vi "USBL_UA TRACKER for boat_rev2.vi"() -> ()   [LabVIEW 2017]
uses:
  <vilib>/Analysis/2dsp.llb/Decimate (single shot, DBL).vi
  <vilib>/DAQmx/read.llb/DAQmx Read (Analog 1D Wfm NChan NSamp).vi
  <vilib>/Analysis/3filter.llb/FIR Filter (DBL).vi
  <vilib>/DAQmx/create/channels.llb/DAQmx Create Channel (AI-Voltage-Basic).vi
  <vilib>/DAQmx/configure/timing.llb/DAQmx Timing (Sample Clock).vi
  <vilib>/DAQmx/miscellaneous.llb/DAQmx Fill In Error Info.vi
  <vilib>/DAQmx/create/channels.llb/DAQmx Create Channel (CO-Pulse Generation-Frequency).vi
  <vilib>/DAQmx/configure/timing.llb/DAQmx Timing (Implicit).vi
  <vilib>/Analysis/NI_AALBase.lvlib
  <vilib>/Analysis/NI_AALPro.lvlib
  <vilib>/Analysis/NI_AAL_SigProc.lvlib
  <resource>/objmgr/daqmx.rc
panel:
  out "Position 7":dbl[](array[numeric])
  out "Position 6":dbl[](array[numeric])
  out "Position 5":dbl[](array[numeric])
  out "Position 4":dbl[](array[numeric])
  out "Position 3":dbl[](array[numeric])
  out "Position 2":dbl[](array[numeric])
  out "Position 1":dbl[](array[numeric])
  out "Position 0":dbl[](array[numeric])
  out "Deci_Chunk":i32
  out "Target code":dbl[](array[numeric])
  out "ThresholdMargin":dbl=10.0
  out "MovingAvrParm":dbl[](array[numeric])
  out "Coefficient_bit1":dbl[](array[numeric])
  out "Coefficient_bit0":dbl[](array[numeric])
  out "Decimation rate":i32=12
  out "Carrier signal":dbl[](array[numeric])
  out "숫자형 7":dbl=7.0
  out "숫자형 6":dbl=7.0
  out "숫자형 5":dbl=7.0
  in  "Number of pulse":i32=160
  in  "Output terminal":tag="/Dev4/PFI0"
  in  "Frequency(Hz)":dbl=32000.0 format="%.6f"
  in  "Cycle share":dbl=0.5 format="%.6f"
  in  "Counter":tag="Dev4/ctr0"
  out "Detect":bool
  in  "User number":i32=12
  out "숫자형 4":dbl=5.0
  out "숫자형 3":dbl=7.0
  out "숫자형 2":dbl=7.0
  out "숫자형":dbl=7.0
  in  "Start frequency(Hz)":dbl format="%#_6p"
  in  "Stop frequency(Hz)":dbl=4000.0 format="%#_6p"
  in  "Symbol length(sec)":dbl=0.128 format="%#_6p"
  in  "Number of sample":i32=38400
  in  "Sampling freuqncy(Hz)":dbl=192000.0 format="%#_6p"
  in  "Physical channel":tag="Dev4/ai0:7" caption="Physical Channel"
  in  "Device":tag="Dev4"
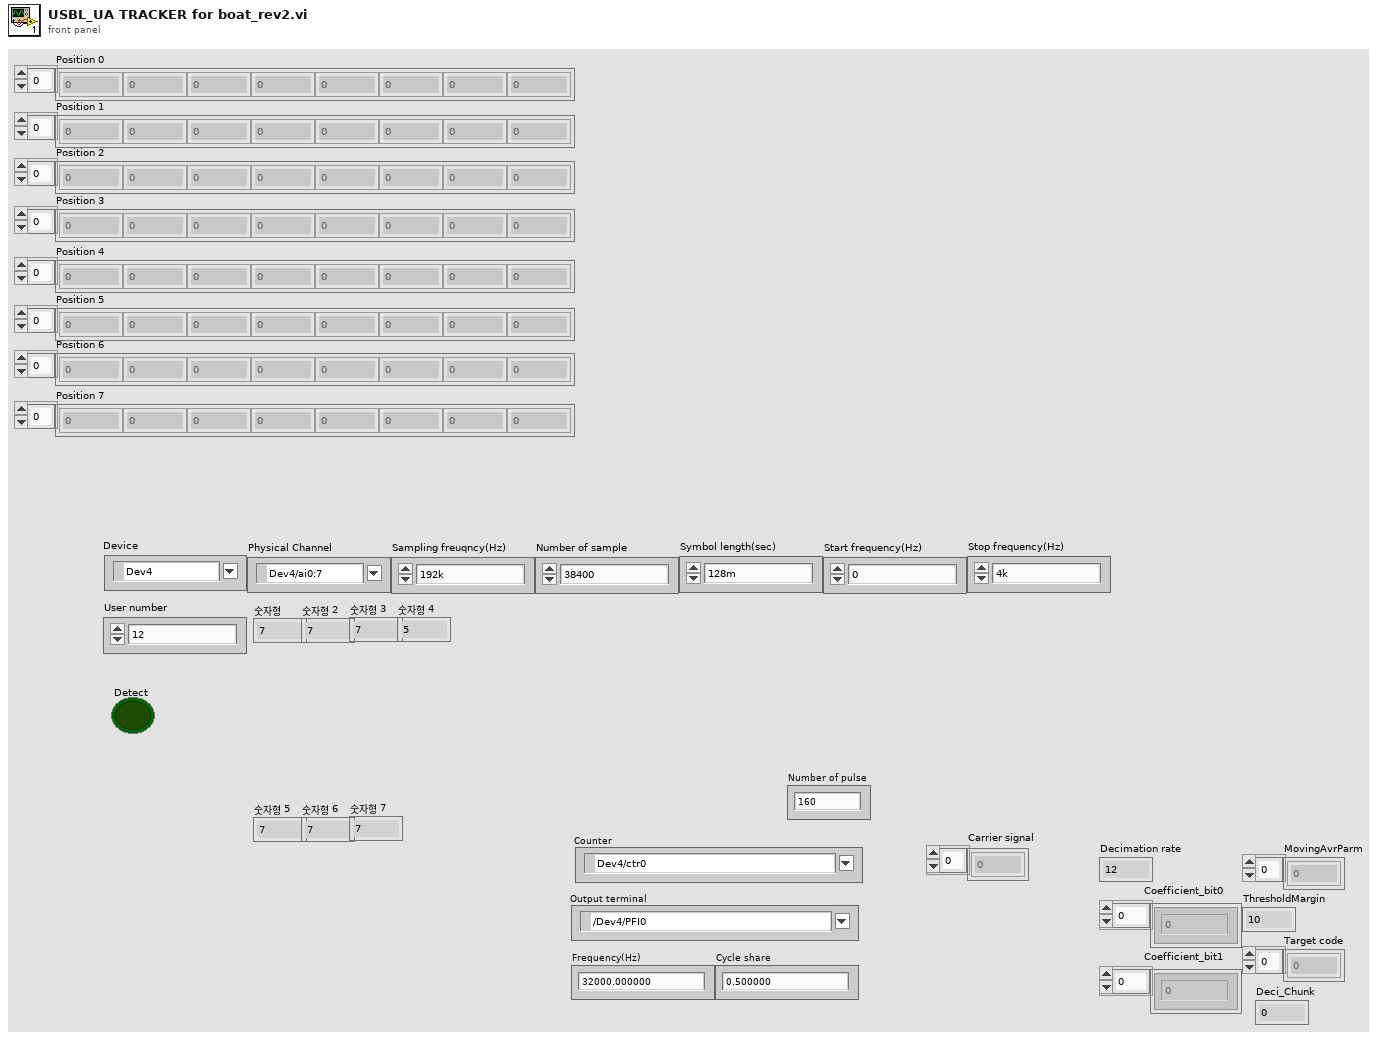
[diagram p1: front panel]
diagram:
  n1 = flat-sequence {
    tunnel: ["Number of sample"] -> w12
    tunnel: [w39] -> w11
    tunnel: ["Sampling freuqncy(Hz)"] -> w10
    tunnel: ["Physical channel"] -> w9
    tunnel: ["Device"] -> w8
    tunnel: [w35] -> w7
    tunnel: [w31] -> w6
    tunnel: [w30] -> w5
    tunnel: [w25] -> w4
    tunnel: [w21] -> w3
    tunnel: [w20] -> w2
    tunnel: [w13] -> w1
    tunnel: w12 -> [w59]
    tunnel: w11 -> [w58]
    tunnel: w10 -> [w57]
    tunnel: w9 -> [w56]
    tunnel: w8 -> [w55]
    tunnel: w7 -> [w54]
    tunnel: w6 -> [w53]
    tunnel: w5 -> [w52]
    tunnel: w4 -> [w49]
    tunnel: w3 -> [w47]
    tunnel: w2 -> [w46]
    tunnel: w1 -> [w43]
    frame #0 {
      w20 = 10.0 ("값")
      w22 = 160 ("차원 크기")
      w35 = 12 ("Divide by")
      w39 = 10123 items=["유한 샘플"=10178, "연속 샘플"=10123, "하드웨어 타이밍에 의한 단일 포인트"=12522] ("sample mode")
      # "Signal gen. (Counter)"
      # "Target code"
      # "EOF"
      # "SOF"
      # "Processing parameter"
      # "Freqeuncy 2"
      # "Freqeuncy 1"
      # "Symbol length"
      # "Moving average window size"
      # "Threshold Margin"
      # "DAQ device setting"
      # "Device"
      # "Physical channel"
      # "Sampling frequency"
      # "Sample mode"
      # "Number of samples per channel"
      n2 = To Double Precision Float(number=w35) -> (double precision float=w41:dbl)
      n3 = To Double Precision Float(number=w22) -> (double precision float=w24:dbl)
      n4 = Divide(x="Sampling freuqncy(Hz)", y=w41) -> (x/y=w29:dbl)
      n5 = Format Into String(format string="%04b" ("포맷 문자열"), "User number") -> (resulting string=w17:string)  [unwired: 2 in, 1 out]
      n6 = Reciprocal(x=w24) -> (1/x=w23:dbl)
      n7 = call "CodeConvert(SubVI).vi"("Code"=w17) -> ("Code_array"=w15:dbl[])
      n8 = Divide(x=30000.0, y="Sampling freuqncy(Hz)") -> (x/y=w33:dbl)
      n9 = Initialize Array(w23, w22) -> (w21:dbl[])
      "MovingAvrParm" <- w21
      n10 = call "ChirpSourceGen(SubVI).vi"("Frequency2(Hz)"="Stop frequency(Hz)", "Frequency1(Hz)"="Start frequency(Hz)", "Pulse length(sec)"="Symbol length(sec)", "Fs(Hz)"=w29) -> ("M.F. Tap(F2-1)"=w25:dbl[], "M.F. Tap(F1-2)"=w31:dbl[])  [unwired: 1 out]
      "Coefficient_bit0" <- w31
      "Coefficient_bit1" <- w25
      n11 = Insert Into Array(array=dbl[] [0.0, 1.0], new element #1=w15, new element #2=dbl[] [1.0, 0.0]) -> (w13:dbl[])  [unwired: 1 in]
      "Target code" <- w13
      n12 = call <vilib>:"Sine Wave.vi"("samples"="Number of sample", "amplitude"=5.0, "frequency"=w33) -> ("sine wave"=w30:dbl[])  [unwired: 2 in, 2 out]
      "Carrier signal" <- w30
      "Decimation rate" <- w35
      "ThresholdMargin" <- w20
    }
    frame #1 {
      n13 = flat-sequence {
        tunnel: w55 -> [w78]
        tunnel: [w79] -> w66
        tunnel: w56 -> [w77]
        tunnel: [w77] -> w65
        tunnel: w57 -> [w75]
        tunnel: [w75] -> w64
        tunnel: w59 -> [w74]
        tunnel: [w74] -> w63
        tunnel: w58 -> [w76]
        tunnel: [w76] -> w62
        tunnel: [w72] -> w61
        tunnel: [w73] -> w60
        tunnel: w54 -> [w73]
        tunnel: w53 -> [w72]
        tunnel: w52 -> [w71]
        tunnel: [w71] -> w51
        tunnel: [w70] -> w50
        tunnel: w49 -> [w70]
        tunnel: [w69] -> w48
        tunnel: w47 -> [w69]
        tunnel: w46 -> [w68]
        tunnel: [w68] -> w45
        tunnel: [w67] -> w44
        tunnel: w43 -> [w67]
        tunnel: w66 -> [w129]
        tunnel: w65 -> [w128]
        tunnel: w64 -> [w127]
        tunnel: w63 -> [w125]
        tunnel: w62 -> [w126]
        tunnel: w61 -> [w114]
        tunnel: w60 -> [w102]
        tunnel: w51 -> [w103]
        tunnel: w50 -> [w87]
        tunnel: w48 -> [w94]
        tunnel: w45 -> [w93]
        tunnel: w44 -> [w88]
        tunnel: [w445] -> w42
        tunnel: w42 -> [w548]
        frame #0 {
          n14 = call <vilib>:"DAQmx Reset Device.vi"("device in"=w78) -> ("error out"=w79:errorcluster)  [unwired: 1 in, 13 out]
        }
        frame #1 {
          w86 = dbl[][] [[-1.0, -1.0, -1.0, -1.0, -1.0, -1.0, -1.0, -1.0], [-1.0, -1.0, -1.0, -1.0, -1.0, -1.0, -1.0, -1.0]]
          w100 = "Proc1" ("이름(이름없음)")
          w101 = "Proc0" ("이름(이름없음)")
          w99 = dbl[][] []
          w115 = "SIG0" ("이름(이름없음)")
          w122 = waveform(dbl) {"t0"=timestamp(0 s since 1904-01-01), "dt"=1.0, "Y"=[]} ("Waveform")
          w105 = "SIG1" ("이름(이름없음)")
          # "Target code"
          # "[Post processing]  1. Queue get : Proc0, Proc1 / 2. Threshold estimation with moving average / 3. Peak and valley detection / 4. Signal detection using time difference of symbol / 5. Demodulation"
          # "[Signal processing]\n1. Queue get : SIG0\n2. Data type converting : Waveform (DBL) --> Array (DBL)\n3. DDC (Digital to Digital Convering)\n  - DSB modulation : Multiply carrier signal (30kHz)\n  - Decimate : 192kHz sample rate --> 16kHz sample rate\n4. Cross-correlation with down-chirp (4k ~ 0Hz)\n5. Envelope detection (Hilbert transform) & square\n6. Queue put : Proc1"
          # "[Signal processing]\n1. Queue get : SIG0\n2. Data type converting : Waveform (DBL) --> Array (DBL)\n3. DDC (Digital to Digital Convering)\n  - DSB modulation : Multiply carrier signal (30kHz)\n  - Decimate : 192kHz sample rate --> 16kHz sample rate\n4. Cross-correlation with up-chirp (0 ~ 4kHz)\n5. Envelope detection (Hilbert transform) & square\n6. Queue put : Proc0"
          # "[Data Acquistion (ADC)]\n1. Device reset\n2. Creat channel\n3, Set sample clock\n  - Sampling frequency : 192kHz\n  - Number of sample (Chunk size) : 38400\n4. Start task\n5. Data read\n6. Queue put : SIG0, SIG1\n  - Queue data type : Waveform (DBL)"
          # "Moving average prameter based on FIR filter calculation"
          # "Coefficient for bit 1 : Down-chirp"
          # "Coefficient for bit 0 : Up-chirp"
          # "Decimation rate"
          # "Carrier signal"
          n15 = call-poly <vilib>:"DAQmx Create Virtual Channel.vi"("physical channels"=w128, "error in"=w129) -> ("task out"=w131:refnum<k21>, "error out"=w130:errorcluster)  [unwired: 7 in, 5 out]
          n16 = call-poly <vilib>:"DAQmx Timing.vi"("task/channels in"=w131, "sample mode"=w126, "samples per channel"=w125, "rate"=w127, "error in"=w130) -> ("task out"=w132:refnum<k21>, "error out"=w133:errorcluster)  [unwired: 2 in, 7 out]
          n17 = call <vilib>:"DAQmx Start Task.vi"("task/channels in"=w132, "error in"=w133) -> ("task out"=w134:refnum<k21>, "error out"=w135:errorcluster)  [unwired: 12 in]
          n18 = Build Array(w122, w122, w122, w122, w122, w122, w122, w122) -> (w104:waveform(dbl)[])
          n19 = Obtain Queue(name (unnamed)=w105, element data type=w104) -> (queue out=w124:refnum<queue>, error out=w123:errorcluster)  [unwired: 3 in, 1 out]
          n20 = Obtain Queue(name (unnamed)=w115, element data type=w104) -> (queue out=w121:refnum<queue>, error out=w120:errorcluster)  [unwired: 3 in, 1 out]
          n21 = while {
            tunnel: w134 -> [w444]
            tunnel: w135 -> [w443]
            tunnel: [w442] -> w138
            tunnel: [w441] -> w139
            tunnel: w125 -> [w440]
            tunnel: w124 -> [w439]
            tunnel: w123 -> [w438]
            tunnel: w121 -> [w437]
            tunnel: w120 -> [w436]
            i -> [w434]
            stop <- w433 stop-if-true
            n22 = call-poly <vilib>:"DAQmx Read.vi"("task/channels in"=w444, "number of samples per channel"=w440, "error in"=w443) -> ("task out"=w442:refnum<k21>, "data"=w435:waveform(dbl)[], "error out"=w441:errorcluster)  [unwired: 10 out]
            n23 = Enqueue Element(queue=w437, element=w435, error in (no error)=w436) -> ()  [unwired: 1 in, 3 out]
            n24 = Enqueue Element(queue=w439, element=w435, error in (no error)=w438) -> ()  [unwired: 1 in, 3 out]
            n25 = local read "Detect"() -> (w433:bool)
            "숫자형" <- w434
          }
          n26 = call <vilib>:"DAQmx Stop Task.vi"("task/channels in"=w138, "error in"=w139) -> ("task out"=w137:refnum<k21>, "error out"=w136:errorcluster)  [unwired: 12 out]
          n27 = call <vilib>:"DAQmx Clear Task.vi"("task in"=w137, "error in"=w136) -> ()  [unwired: 14 out]
          n28 = Obtain Queue(name (unnamed)=w101, element data type=w99) -> (queue out=w119:refnum<queue>, error out=w118:errorcluster)  [unwired: 3 in, 1 out]
          n29 = Obtain Queue(name (unnamed)=w115, element data type=w104) -> (queue out=w117:refnum<queue>, error out=w116:errorcluster)  [unwired: 3 in, 1 out]
          n30 = while {
            tunnel: w117 -> [w432]
            tunnel: w116 -> [w431]
            tunnel: w119 -> [w430]
            tunnel: w118 -> [w429]
            tunnel: [w428] -> w113
            tunnel: [w427] -> w112
            tunnel: w103 -> [w367]
            tunnel: w102 -> [w366]
            tunnel: w114 -> [w365]
            i -> [w363]
            stop <- w362 stop-if-true
            w377 = TRUE ("averaging")
            w426 = TRUE ("init/cont (init:F)")
            n31 = Dequeue Element(queue=w432, error in (no error)=w431) -> (queue out=w428:refnum<queue>, element=w368:waveform(dbl)[], error out=w427:errorcluster)  [unwired: 2 out]
            n32 = Index Array(array=w368) -> (element #1=w425:waveform(dbl), element #2=w424:waveform(dbl), element #3=w423:waveform(dbl), element #4=w422:waveform(dbl), element #5=w421:waveform(dbl), element #6=w420:waveform(dbl), element #7=w419:waveform(dbl), element #8=w418:waveform(dbl))  [unwired: 8 in]
            n33 = Unbundle By Name(w425) -> ("Y"=w417:dbl[])
            n34 = Unbundle By Name(w424) -> ("Y"=w416:dbl[])
            n35 = Unbundle By Name(w423) -> ("Y"=w415:dbl[])
            n36 = Unbundle By Name(w422) -> ("Y"=w414:dbl[])
            n37 = Unbundle By Name(w421) -> ("Y"=w413:dbl[])
            n38 = Unbundle By Name(w420) -> ("Y"=w412:dbl[])
            n39 = Unbundle By Name(w419) -> ("Y"=w411:dbl[])
            n40 = Unbundle By Name(w418) -> ("Y"=w410:dbl[])
            n41 = Multiply(x=w417, y=w367) -> (x*y=w392:dbl[])
            n42 = Multiply(x=w416, y=w367) -> (x*y=w391:dbl[])
            n43 = Multiply(x=w415, y=w367) -> (x*y=w390:dbl[])
            n44 = Multiply(x=w414, y=w367) -> (x*y=w389:dbl[])
            n45 = Multiply(x=w413, y=w367) -> (x*y=w388:dbl[])
            n46 = Multiply(x=w412, y=w367) -> (x*y=w387:dbl[])
            n47 = Multiply(x=w411, y=w367) -> (x*y=w386:dbl[])
            n48 = Multiply(x=w410, y=w367) -> (x*y=w385:dbl[])
            n49 = call-poly <vilib>:"Decimate (single shot).vi"("averaging"=w377, "decimating factor"=w366, "X"=w387) -> ("Decimated Array"=w380:dbl[])  [unwired: 7 in, 1 out]
            n50 = call-poly <vilib>:"Decimate (single shot).vi"("averaging"=w377, "decimating factor"=w366, "X"=w385) -> ("Decimated Array"=w378:dbl[])  [unwired: 7 in, 1 out]
            n51 = call-poly <vilib>:"Decimate (single shot).vi"("averaging"=w377, "decimating factor"=w366, "X"=w391) -> ("Decimated Array"=w384:dbl[])  [unwired: 7 in, 1 out]
            n52 = call-poly <vilib>:"Decimate (single shot).vi"("averaging"=w377, "decimating factor"=w366, "X"=w389) -> ("Decimated Array"=w382:dbl[])  [unwired: 7 in, 1 out]
            n53 = call-poly <vilib>:"Decimate (single shot).vi"("averaging"=w377, "decimating factor"=w366, "X"=w388) -> ("Decimated Array"=w381:dbl[])  [unwired: 7 in, 1 out]
            n54 = call-poly <vilib>:"Decimate (single shot).vi"("averaging"=w377, "decimating factor"=w366, "X"=w386) -> ("Decimated Array"=w379:dbl[])  [unwired: 7 in, 1 out]
            n55 = call-poly <vilib>:"Decimate (single shot).vi"("averaging"=w377, "decimating factor"=w366, "X"=w392) -> ("Decimated Array"=w393:dbl[])  [unwired: 7 in, 1 out]
            n56 = call-poly <vilib>:"Decimate (single shot).vi"("averaging"=w377, "decimating factor"=w366, "X"=w390) -> ("Decimated Array"=w383:dbl[])  [unwired: 7 in, 1 out]
            n57 = call-poly <vilib>:"FIR Filter.vi"("init/cont (init:F)"=w426, "FIR Coefficients"=w365, "X"=w393) -> ("Filtered X"=w409:dbl[])  [unwired: 1 in, 1 out]
            n58 = call-poly <vilib>:"FIR Filter.vi"("init/cont (init:F)"=w426, "FIR Coefficients"=w365, "X"=w384) -> ("Filtered X"=w408:dbl[])  [unwired: 1 in, 1 out]
            n59 = call-poly <vilib>:"FIR Filter.vi"("init/cont (init:F)"=w426, "FIR Coefficients"=w365, "X"=w383) -> ("Filtered X"=w407:dbl[])  [unwired: 1 in, 1 out]
            n60 = call-poly <vilib>:"FIR Filter.vi"("init/cont (init:F)"=w426, "FIR Coefficients"=w365, "X"=w382) -> ("Filtered X"=w406:dbl[])  [unwired: 1 in, 1 out]
            n61 = call-poly <vilib>:"FIR Filter.vi"("init/cont (init:F)"=w426, "FIR Coefficients"=w365, "X"=w381) -> ("Filtered X"=w405:dbl[])  [unwired: 1 in, 1 out]
            n62 = call-poly <vilib>:"FIR Filter.vi"("init/cont (init:F)"=w426, "FIR Coefficients"=w365, "X"=w380) -> ("Filtered X"=w404:dbl[])  [unwired: 1 in, 1 out]
            n63 = call-poly <vilib>:"FIR Filter.vi"("init/cont (init:F)"=w426, "FIR Coefficients"=w365, "X"=w379) -> ("Filtered X"=w403:dbl[])  [unwired: 1 in, 1 out]
            n64 = call-poly <vilib>:"FIR Filter.vi"("init/cont (init:F)"=w426, "FIR Coefficients"=w365, "X"=w378) -> ("Filtered X"=w402:dbl[])  [unwired: 1 in, 1 out]
            n65 = call "Envelope(SubVI).vi"("x"=w409) -> ("Y"=w401:dbl[])
            n66 = call "Envelope(SubVI).vi"("x"=w408) -> ("Y"=w400:dbl[])
            n67 = call "Envelope(SubVI).vi"("x"=w407) -> ("Y"=w399:dbl[])
            n68 = call "Envelope(SubVI).vi"("x"=w406) -> ("Y"=w398:dbl[])
            n69 = call "Envelope(SubVI).vi"("x"=w405) -> ("Y"=w397:dbl[])
            n70 = call "Envelope(SubVI).vi"("x"=w404) -> ("Y"=w396:dbl[])
            n71 = call "Envelope(SubVI).vi"("x"=w403) -> ("Y"=w395:dbl[])
            n72 = call "Envelope(SubVI).vi"("x"=w402) -> ("Y"=w394:dbl[])
            n73 = Square(x=w401) -> (x^2=w376:dbl[])
            n74 = Square(x=w400) -> (x^2=w375:dbl[])
            n75 = Square(x=w399) -> (x^2=w374:dbl[])
            n76 = Square(x=w398) -> (x^2=w373:dbl[])
            n77 = Square(x=w397) -> (x^2=w372:dbl[])
            n78 = Square(x=w396) -> (x^2=w371:dbl[])
            n79 = Square(x=w395) -> (x^2=w370:dbl[])
            n80 = Square(x=w394) -> (x^2=w369:dbl[])
            n81 = local read "Detect"() -> (w362:bool)
            n82 = Build Array(w376, w375, w374, w373, w372, w371, w370, w369) -> (w364:dbl[][])
            n83 = Enqueue Element(queue=w430, element=w364, error in (no error)=w429) -> ()  [unwired: 1 in, 3 out]
            "숫자형 2" <- w363
          }
          n84 = Release Queue(queue=w113, error in (no error)=w112) -> ()  [unwired: 1 in, 3 out]
          n85 = Obtain Queue(name (unnamed)=w100, element data type=w99) -> (queue out=w111:refnum<queue>, error out=w110:errorcluster)  [unwired: 3 in, 1 out]
          n86 = Obtain Queue(name (unnamed)=w105, element data type=w104) -> (queue out=w109:refnum<queue>, error out=w108:errorcluster)  [unwired: 3 in, 1 out]
          n87 = while {
            tunnel: w109 -> [w361]
            tunnel: w108 -> [w360]
            tunnel: w111 -> [w359]
            tunnel: w110 -> [w358]
            tunnel: [w357] -> w107
            tunnel: [w356] -> w106
            tunnel: w103 -> [w296]
            tunnel: w102 -> [w295]
            tunnel: w87 -> [w294]
            i -> [w292]
            stop <- w291 stop-if-true
            w306 = TRUE ("averaging")
            w355 = TRUE ("init/cont (init:F)")
            n88 = Dequeue Element(queue=w361, error in (no error)=w360) -> (queue out=w357:refnum<queue>, element=w297:waveform(dbl)[], error out=w356:errorcluster)  [unwired: 2 out]
            n89 = Index Array(array=w297) -> (element #1=w354:waveform(dbl), element #2=w353:waveform(dbl), element #3=w352:waveform(dbl), element #4=w351:waveform(dbl), element #5=w350:waveform(dbl), element #6=w349:waveform(dbl), element #7=w348:waveform(dbl), element #8=w347:waveform(dbl))  [unwired: 8 in]
            n90 = Unbundle By Name(w354) -> ("Y"=w346:dbl[])
            n91 = Unbundle By Name(w353) -> ("Y"=w345:dbl[])
            n92 = Unbundle By Name(w352) -> ("Y"=w344:dbl[])
            n93 = Unbundle By Name(w351) -> ("Y"=w343:dbl[])
            n94 = Unbundle By Name(w350) -> ("Y"=w342:dbl[])
            n95 = Unbundle By Name(w349) -> ("Y"=w341:dbl[])
            n96 = Unbundle By Name(w348) -> ("Y"=w340:dbl[])
            n97 = Unbundle By Name(w347) -> ("Y"=w339:dbl[])
            n98 = Multiply(x=w346, y=w296) -> (x*y=w321:dbl[])
            n99 = Multiply(x=w345, y=w296) -> (x*y=w320:dbl[])
            n100 = Multiply(x=w344, y=w296) -> (x*y=w319:dbl[])
            n101 = Multiply(x=w343, y=w296) -> (x*y=w318:dbl[])
            n102 = Multiply(x=w342, y=w296) -> (x*y=w317:dbl[])
            n103 = Multiply(x=w341, y=w296) -> (x*y=w316:dbl[])
            n104 = Multiply(x=w340, y=w296) -> (x*y=w315:dbl[])
            n105 = Multiply(x=w339, y=w296) -> (x*y=w314:dbl[])
            n106 = call-poly <vilib>:"Decimate (single shot).vi"("averaging"=w306, "decimating factor"=w295, "X"=w316) -> ("Decimated Array"=w309:dbl[])  [unwired: 7 in, 1 out]
            n107 = call-poly <vilib>:"Decimate (single shot).vi"("averaging"=w306, "decimating factor"=w295, "X"=w314) -> ("Decimated Array"=w307:dbl[])  [unwired: 7 in, 1 out]
            n108 = call-poly <vilib>:"Decimate (single shot).vi"("averaging"=w306, "decimating factor"=w295, "X"=w320) -> ("Decimated Array"=w313:dbl[])  [unwired: 7 in, 1 out]
            n109 = call-poly <vilib>:"Decimate (single shot).vi"("averaging"=w306, "decimating factor"=w295, "X"=w318) -> ("Decimated Array"=w311:dbl[])  [unwired: 7 in, 1 out]
            n110 = call-poly <vilib>:"Decimate (single shot).vi"("averaging"=w306, "decimating factor"=w295, "X"=w317) -> ("Decimated Array"=w310:dbl[])  [unwired: 7 in, 1 out]
            n111 = call-poly <vilib>:"Decimate (single shot).vi"("averaging"=w306, "decimating factor"=w295, "X"=w315) -> ("Decimated Array"=w308:dbl[])  [unwired: 7 in, 1 out]
            n112 = call-poly <vilib>:"Decimate (single shot).vi"("averaging"=w306, "decimating factor"=w295, "X"=w321) -> ("Decimated Array"=w322:dbl[])  [unwired: 7 in, 1 out]
            n113 = call-poly <vilib>:"Decimate (single shot).vi"("averaging"=w306, "decimating factor"=w295, "X"=w319) -> ("Decimated Array"=w312:dbl[])  [unwired: 7 in, 1 out]
            n114 = call-poly <vilib>:"FIR Filter.vi"("init/cont (init:F)"=w355, "FIR Coefficients"=w294, "X"=w322) -> ("Filtered X"=w338:dbl[])  [unwired: 1 in, 1 out]
            n115 = call-poly <vilib>:"FIR Filter.vi"("init/cont (init:F)"=w355, "FIR Coefficients"=w294, "X"=w313) -> ("Filtered X"=w337:dbl[])  [unwired: 1 in, 1 out]
            n116 = call-poly <vilib>:"FIR Filter.vi"("init/cont (init:F)"=w355, "FIR Coefficients"=w294, "X"=w312) -> ("Filtered X"=w336:dbl[])  [unwired: 1 in, 1 out]
            n117 = call-poly <vilib>:"FIR Filter.vi"("init/cont (init:F)"=w355, "FIR Coefficients"=w294, "X"=w311) -> ("Filtered X"=w335:dbl[])  [unwired: 1 in, 1 out]
            n118 = call-poly <vilib>:"FIR Filter.vi"("init/cont (init:F)"=w355, "FIR Coefficients"=w294, "X"=w310) -> ("Filtered X"=w334:dbl[])  [unwired: 1 in, 1 out]
            n119 = call-poly <vilib>:"FIR Filter.vi"("init/cont (init:F)"=w355, "FIR Coefficients"=w294, "X"=w309) -> ("Filtered X"=w333:dbl[])  [unwired: 1 in, 1 out]
            n120 = call-poly <vilib>:"FIR Filter.vi"("init/cont (init:F)"=w355, "FIR Coefficients"=w294, "X"=w308) -> ("Filtered X"=w332:dbl[])  [unwired: 1 in, 1 out]
            n121 = call-poly <vilib>:"FIR Filter.vi"("init/cont (init:F)"=w355, "FIR Coefficients"=w294, "X"=w307) -> ("Filtered X"=w331:dbl[])  [unwired: 1 in, 1 out]
            n122 = call "Envelope(SubVI).vi"("x"=w338) -> ("Y"=w330:dbl[])
            n123 = call "Envelope(SubVI).vi"("x"=w337) -> ("Y"=w329:dbl[])
            n124 = call "Envelope(SubVI).vi"("x"=w336) -> ("Y"=w328:dbl[])
            n125 = call "Envelope(SubVI).vi"("x"=w335) -> ("Y"=w327:dbl[])
            n126 = call "Envelope(SubVI).vi"("x"=w334) -> ("Y"=w326:dbl[])
            n127 = call "Envelope(SubVI).vi"("x"=w333) -> ("Y"=w325:dbl[])
            n128 = call "Envelope(SubVI).vi"("x"=w332) -> ("Y"=w324:dbl[])
            n129 = call "Envelope(SubVI).vi"("x"=w331) -> ("Y"=w323:dbl[])
            n130 = Square(x=w330) -> (x^2=w305:dbl[])
            n131 = Square(x=w329) -> (x^2=w304:dbl[])
            n132 = Square(x=w328) -> (x^2=w303:dbl[])
            n133 = Square(x=w327) -> (x^2=w302:dbl[])
            n134 = Square(x=w326) -> (x^2=w301:dbl[])
            n135 = Square(x=w325) -> (x^2=w300:dbl[])
            n136 = Square(x=w324) -> (x^2=w299:dbl[])
            n137 = Square(x=w323) -> (x^2=w298:dbl[])
            n138 = local read "Detect"() -> (w291:bool)
            n139 = Build Array(w305, w304, w303, w302, w301, w300, w299, w298) -> (w293:dbl[][])
            n140 = Enqueue Element(queue=w359, element=w293, error in (no error)=w358) -> ()  [unwired: 1 in, 3 out]
            "숫자형 3" <- w292
          }
          n141 = local read "Number of sample"() -> (w85:i32)
          n142 = local read "Decimation rate"() -> (w81:i32)
          n143 = To Double Precision Float(number=w81) -> (double precision float=w80:dbl)
          n144 = To Double Precision Float(number=w85) -> (double precision float=w84:dbl)
          n145 = Divide(x=w84, y=w80) -> (x/y=w83:dbl)
          n146 = To Long Integer(number=w83) -> (32bit integer=w82:i32)
          "Deci_Chunk" <- w82
          n147 = Release Queue(queue=w107, error in (no error)=w106) -> ()  [unwired: 1 in, 3 out]
          n148 = Obtain Queue(name (unnamed)=w101, element data type=w99) -> (queue out=w98:refnum<queue>, error out=w97:errorcluster)  [unwired: 3 in, 1 out]
          n149 = Obtain Queue(name (unnamed)=w100, element data type=w99) -> (queue out=w96:refnum<queue>, error out=w95:errorcluster)  [unwired: 3 in, 1 out]
          n150 = while {
            tunnel: w98 -> [w290]
            tunnel: w97 -> [w289]
            tunnel: w96 -> [w288]
            tunnel: w95 -> [w287]
            tunnel: w94 -> [w285]
            tunnel: w93 -> [w249]
            tunnel: [w229] -> w92
            tunnel: [w228] -> w91
            tunnel: [w227] -> w90
            tunnel: [w226] -> w89
            tunnel: w88 -> [w225]
            shift-right: [w140] -> _
            shift-left: w86 -> [w163]
            shift-right: [w141] -> _
            shift-left: w86 -> [w162]
            shift-right: [w142] -> _
            shift-left: w86 -> [w161]
            shift-right: [w143] -> _
            shift-left: w86 -> [w160]
            shift-right: [w144] -> _
            shift-left: w86 -> [w159]
            shift-right: [w145] -> _
            shift-left: w86 -> [w158]
            shift-right: [w146] -> _
            shift-left: w86 -> [w157]
            shift-right: [w147] -> _
            shift-left: w86 -> [w156]
            tunnel: w82 -> [w181]
            i -> [w180]
            stop <- w214 stop-if-true
            w274 = enum32{"Peaks", "Valleys"}."Valleys" ("peaks/valleys")
            w275 = enum32{"Peaks", "Valleys"}."Peaks" ("peaks/valleys")
            w273 = 5 ("width")
            w284 = TRUE ("init/cont (init:F)")
            n151 = Dequeue Element(queue=w290, error in (no error)=w289) -> (queue out=w229:refnum<queue>, element=w231:dbl[][], error out=w228:errorcluster)  [unwired: 2 out]
            n152 = Dequeue Element(queue=w288, error in (no error)=w287) -> (queue out=w227:refnum<queue>, element=w230:dbl[][], error out=w226:errorcluster)  [unwired: 2 out]
            n153 = Subtract(x=w231, y=w230) -> (x-y=w286:dbl[][])
            n154 = Index Array(array=w286) -> (element #1=w272:dbl[], element #2=w271:dbl[], element #3=w270:dbl[], element #4=w269:dbl[], element #5=w268:dbl[], element #6=w267:dbl[], element #7=w266:dbl[], element #8=w234:dbl[])  [unwired: 16 in]
            n155 = call-poly <vilib>:"FIR Filter.vi"("init/cont (init:F)"=w284, "FIR Coefficients"=w285, "X"=w272) -> ("Filtered X"=w283:dbl[])  [unwired: 1 in, 1 out]
            n156 = call-poly <vilib>:"FIR Filter.vi"("init/cont (init:F)"=w284, "FIR Coefficients"=w285, "X"=w271) -> ("Filtered X"=w282:dbl[])  [unwired: 1 in, 1 out]
            n157 = call-poly <vilib>:"FIR Filter.vi"("init/cont (init:F)"=w284, "FIR Coefficients"=w285, "X"=w270) -> ("Filtered X"=w281:dbl[])  [unwired: 1 in, 1 out]
            n158 = call-poly <vilib>:"FIR Filter.vi"("init/cont (init:F)"=w284, "FIR Coefficients"=w285, "X"=w269) -> ("Filtered X"=w280:dbl[])  [unwired: 1 in, 1 out]
            n159 = call-poly <vilib>:"FIR Filter.vi"("init/cont (init:F)"=w284, "FIR Coefficients"=w285, "X"=w268) -> ("Filtered X"=w279:dbl[])  [unwired: 1 in, 1 out]
            n160 = call-poly <vilib>:"FIR Filter.vi"("init/cont (init:F)"=w284, "FIR Coefficients"=w285, "X"=w267) -> ("Filtered X"=w278:dbl[])  [unwired: 1 in, 1 out]
            n161 = call-poly <vilib>:"FIR Filter.vi"("init/cont (init:F)"=w284, "FIR Coefficients"=w285, "X"=w266) -> ("Filtered X"=w277:dbl[])  [unwired: 1 in, 1 out]
            n162 = call-poly <vilib>:"FIR Filter.vi"("init/cont (init:F)"=w284, "FIR Coefficients"=w285, "X"=w234) -> ("Filtered X"=w276:dbl[])  [unwired: 1 in, 1 out]
            n163 = Array Max & Min(array=w283) -> (max value=w265:dbl, min value=w264:dbl)  [unwired: 2 out]
            n164 = Array Max & Min(array=w282) -> (max value=w263:dbl, min value=w262:dbl)  [unwired: 2 out]
            n165 = Array Max & Min(array=w281) -> (max value=w261:dbl, min value=w260:dbl)  [unwired: 2 out]
            n166 = Array Max & Min(array=w280) -> (max value=w259:dbl, min value=w258:dbl)  [unwired: 2 out]
            n167 = Array Max & Min(array=w279) -> (max value=w257:dbl, min value=w256:dbl)  [unwired: 2 out]
            n168 = Array Max & Min(array=w278) -> (max value=w255:dbl, min value=w254:dbl)  [unwired: 2 out]
            n169 = Array Max & Min(array=w277) -> (max value=w253:dbl, min value=w252:dbl)  [unwired: 2 out]
            n170 = Array Max & Min(array=w276) -> (max value=w251:dbl, min value=w250:dbl)  [unwired: 2 out]
            n171 = call "ThresholdEstimation(SubVI).vi"("Margin"=w249, "최소값"=w262, "최대값"=w263) -> ("N.Th"=w236:dbl, "P.Th"=w247:dbl)
            n172 = call "ThresholdEstimation(SubVI).vi"("Margin"=w249, "최소값"=w260, "최대값"=w261) -> ("N.Th"=w237:dbl, "P.Th"=w246:dbl)
            n173 = call "ThresholdEstimation(SubVI).vi"("Margin"=w249, "최소값"=w258, "최대값"=w259) -> ("N.Th"=w238:dbl, "P.Th"=w245:dbl)
            n174 = call "ThresholdEstimation(SubVI).vi"("Margin"=w249, "최소값"=w256, "최대값"=w257) -> ("N.Th"=w239:dbl, "P.Th"=w244:dbl)
            n175 = call "ThresholdEstimation(SubVI).vi"("Margin"=w249, "최소값"=w264, "최대값"=w265) -> ("N.Th"=w235:dbl, "P.Th"=w248:dbl)
            n176 = call "ThresholdEstimation(SubVI).vi"("Margin"=w249, "최소값"=w254, "최대값"=w255) -> ("N.Th"=w240:dbl, "P.Th"=w243:dbl)
            n177 = call "ThresholdEstimation(SubVI).vi"("Margin"=w249, "최소값"=w252, "최대값"=w253) -> ("N.Th"=w241:dbl, "P.Th"=w242:dbl)
            n178 = call "ThresholdEstimation(SubVI).vi"("Margin"=w249, "최소값"=w250, "최대값"=w251) -> ("N.Th"=w233:dbl, "P.Th"=w232:dbl)
            n179 = call <vilib>:"Peak Detector.vi"("peaks/valleys"=w275, "width"=w273, "threshold"=w248, "X"=w272) -> ("Locations"=w211:dbl[], "# found"=w213:i32)  [unwired: 3 in, 3 out]
            n180 = call <vilib>:"Peak Detector.vi"("peaks/valleys"=w275, "width"=w273, "threshold"=w247, "X"=w271) -> ("Locations"=w207:dbl[], "# found"=w209:i32)  [unwired: 3 in, 3 out]
            n181 = call <vilib>:"Peak Detector.vi"("peaks/valleys"=w275, "width"=w273, "threshold"=w246, "X"=w270) -> ("Locations"=w203:dbl[], "# found"=w205:i32)  [unwired: 3 in, 3 out]
            n182 = call <vilib>:"Peak Detector.vi"("peaks/valleys"=w275, "width"=w273, "threshold"=w245, "X"=w269) -> ("Locations"=w199:dbl[], "# found"=w201:i32)  [unwired: 3 in, 3 out]
            n183 = call <vilib>:"Peak Detector.vi"("peaks/valleys"=w275, "width"=w273, "threshold"=w244, "X"=w268) -> ("Locations"=w195:dbl[], "# found"=w197:i32)  [unwired: 3 in, 3 out]
            n184 = call <vilib>:"Peak Detector.vi"("peaks/valleys"=w275, "width"=w273, "threshold"=w243, "X"=w267) -> ("Locations"=w191:dbl[], "# found"=w193:i32)  [unwired: 3 in, 3 out]
            n185 = call <vilib>:"Peak Detector.vi"("peaks/valleys"=w275, "width"=w273, "threshold"=w242, "X"=w266) -> ("Locations"=w187:dbl[], "# found"=w189:i32)  [unwired: 3 in, 3 out]
            n186 = call <vilib>:"Peak Detector.vi"("peaks/valleys"=w275, "width"=w273, "threshold"=w232, "X"=w234) -> ("Locations"=w183:dbl[], "# found"=w185:i32)  [unwired: 3 in, 3 out]
            n187 = call <vilib>:"Peak Detector.vi"("peaks/valleys"=w274, "width"=w273, "threshold"=w235, "X"=w272) -> ("Locations"=w210:dbl[], "# found"=w212:i32)  [unwired: 3 in, 3 out]
            n188 = call <vilib>:"Peak Detector.vi"("peaks/valleys"=w274, "width"=w273, "threshold"=w236, "X"=w271) -> ("Locations"=w206:dbl[], "# found"=w208:i32)  [unwired: 3 in, 3 out]
            n189 = call <vilib>:"Peak Detector.vi"("peaks/valleys"=w274, "width"=w273, "threshold"=w237, "X"=w270) -> ("Locations"=w202:dbl[], "# found"=w204:i32)  [unwired: 3 in, 3 out]
            n190 = call <vilib>:"Peak Detector.vi"("peaks/valleys"=w274, "width"=w273, "threshold"=w238, "X"=w269) -> ("Locations"=w198:dbl[], "# found"=w200:i32)  [unwired: 3 in, 3 out]
            n191 = call <vilib>:"Peak Detector.vi"("peaks/valleys"=w274, "width"=w273, "threshold"=w239, "X"=w268) -> ("Locations"=w194:dbl[], "# found"=w196:i32)  [unwired: 3 in, 3 out]
            n192 = call <vilib>:"Peak Detector.vi"("peaks/valleys"=w274, "width"=w273, "threshold"=w240, "X"=w267) -> ("Locations"=w190:dbl[], "# found"=w192:i32)  [unwired: 3 in, 3 out]
            n193 = call <vilib>:"Peak Detector.vi"("peaks/valleys"=w274, "width"=w273, "threshold"=w241, "X"=w266) -> ("Locations"=w186:dbl[], "# found"=w188:i32)  [unwired: 3 in, 3 out]
            n194 = call <vilib>:"Peak Detector.vi"("peaks/valleys"=w274, "width"=w273, "threshold"=w233, "X"=w234) -> ("Locations"=w182:dbl[], "# found"=w184:i32)  [unwired: 3 in, 3 out]
            n195 = call "Decision2(SubVI).vi"("L_ind0"=w213, "number of sample"=w181, "L_ind1"=w212, "Peak_ind0"=w211, "index"=w180, "Peak_ind1"=w210) -> ("L_sum"=w148:i32, "Bits"=w179:dbl[], "Position"=w178:dbl[])
            n196 = call "Decision2(SubVI).vi"("L_ind0"=w209, "number of sample"=w181, "L_ind1"=w208, "Peak_ind0"=w207, "index"=w180, "Peak_ind1"=w206) -> ("L_sum"=w149:i32, "Bits"=w177:dbl[], "Position"=w176:dbl[])
            n197 = call "Decision2(SubVI).vi"("L_ind0"=w205, "number of sample"=w181, "L_ind1"=w204, "Peak_ind0"=w203, "index"=w180, "Peak_ind1"=w202) -> ("L_sum"=w150:i32, "Bits"=w175:dbl[], "Position"=w174:dbl[])
            n198 = call "Decision2(SubVI).vi"("L_ind0"=w201, "number of sample"=w181, "L_ind1"=w200, "Peak_ind0"=w199, "index"=w180, "Peak_ind1"=w198) -> ("L_sum"=w151:i32, "Bits"=w173:dbl[], "Position"=w172:dbl[])
            n199 = call "Decision2(SubVI).vi"("L_ind0"=w197, "number of sample"=w181, "L_ind1"=w196, "Peak_ind0"=w195, "index"=w180, "Peak_ind1"=w194) -> ("L_sum"=w152:i32, "Bits"=w171:dbl[], "Position"=w170:dbl[])
            n200 = call "Decision2(SubVI).vi"("L_ind0"=w193, "number of sample"=w181, "L_ind1"=w192, "Peak_ind0"=w191, "index"=w180, "Peak_ind1"=w190) -> ("L_sum"=w153:i32, "Bits"=w169:dbl[], "Position"=w168:dbl[])
            n201 = call "Decision2(SubVI).vi"("L_ind0"=w189, "number of sample"=w181, "L_ind1"=w188, "Peak_ind0"=w187, "index"=w180, "Peak_ind1"=w186) -> ("L_sum"=w154:i32, "Bits"=w167:dbl[], "Position"=w166:dbl[])
            n202 = call "Decision2(SubVI).vi"("L_ind0"=w185, "number of sample"=w181, "L_ind1"=w184, "Peak_ind0"=w183, "index"=w180, "Peak_ind1"=w182) -> ("L_sum"=w155:i32, "Bits"=w165:dbl[], "Position"=w164:dbl[])
            n203 = call "TImeThresholdLogic(SubVI).vi"("Position"=w178, "Bits"=w179, "Buffer"=w163) -> ("Data"=w140:dbl[][])  [unwired: 1 in]
            n204 = call "TImeThresholdLogic(SubVI).vi"("Position"=w176, "Bits"=w177, "Buffer"=w162) -> ("Data"=w141:dbl[][])  [unwired: 1 in]
            n205 = call "TImeThresholdLogic(SubVI).vi"("Position"=w174, "Bits"=w175, "Buffer"=w161) -> ("Data"=w142:dbl[][])  [unwired: 1 in]
            n206 = call "TImeThresholdLogic(SubVI).vi"("Position"=w172, "Bits"=w173, "Buffer"=w160) -> ("Data"=w143:dbl[][])  [unwired: 1 in]
            n207 = call "TImeThresholdLogic(SubVI).vi"("Position"=w170, "Bits"=w171, "Buffer"=w159) -> ("Data"=w144:dbl[][])  [unwired: 1 in]
            n208 = call "TImeThresholdLogic(SubVI).vi"("Position"=w168, "Bits"=w169, "Buffer"=w158) -> ("Data"=w145:dbl[][])  [unwired: 1 in]
            n209 = call "TImeThresholdLogic(SubVI).vi"("Position"=w166, "Bits"=w167, "Buffer"=w157) -> ("Data"=w146:dbl[][])  [unwired: 1 in]
            n210 = call "TImeThresholdLogic(SubVI).vi"("Position"=w164, "Bits"=w165, "Buffer"=w156) -> ("Data"=w147:dbl[][])  [unwired: 1 in]
            n211 = call "CodeDetection(SubVI).vi"("Code"=w225, "Buff"=w140, "L_sum"=w148) -> ("detect"=w224:bool)  [unwired: 1 out]
            n212 = call "CodeDetection(SubVI).vi"("Code"=w225, "Buff"=w141, "L_sum"=w149) -> ("detect"=w223:bool)  [unwired: 1 out]
            n213 = call "CodeDetection(SubVI).vi"("Code"=w225, "Buff"=w142, "L_sum"=w150) -> ("detect"=w222:bool)  [unwired: 1 out]
            n214 = call "CodeDetection(SubVI).vi"("Code"=w225, "Buff"=w143, "L_sum"=w151) -> ("detect"=w221:bool)  [unwired: 1 out]
            n215 = call "CodeDetection(SubVI).vi"("Code"=w225, "Buff"=w144, "L_sum"=w152) -> ("detect"=w220:bool)  [unwired: 1 out]
            n216 = call "CodeDetection(SubVI).vi"("Code"=w225, "Buff"=w145, "L_sum"=w153) -> ("detect"=w219:bool)  [unwired: 1 out]
            n217 = call "CodeDetection(SubVI).vi"("Code"=w225, "Buff"=w146, "L_sum"=w154) -> ("detect"=w218:bool)  [unwired: 1 out]
            n218 = call "CodeDetection(SubVI).vi"("Code"=w225, "Buff"=w147, "L_sum"=w155) -> ("detect"=w217:bool)  [unwired: 1 out]
            n219 = Build Array(w224, w223, w222, w221, w220, w219, w218, w217) -> (w216:bool[])
            n220 = Boolean Array To Number(Boolean array=w216) -> (number=w215:u32)
            n221 = Greater Than 0?(x=w215) -> (x > 0?=w214:bool)
            "Detect" <- w214
            "숫자형 4" <- w180
          }
          n222 = Release Queue(queue=w92, error in (no error)=w91) -> ()  [unwired: 1 in, 3 out]
          n223 = Release Queue(queue=w90, error in (no error)=w89) -> ()  [unwired: 1 in, 3 out]
        }
        frame #2 {
          n224 = local read "Device"() -> (w446:tag)
          n225 = call <vilib>:"DAQmx Reset Device.vi"("device in"=w446) -> ("error out"=w445:errorcluster)  [unwired: 1 in, 13 out]
        }
        frame #3 {
          w447 = dbl[] []
          w456 = dbl[][] [[-1.0, -1.0, -1.0, -1.0, -1.0, -1.0, -1.0, -1.0], [-1.0, -1.0, -1.0, -1.0, -1.0, -1.0, -1.0, -1.0]]
          w475 = dbl[][] []
          w491 = waveform(dbl) {"t0"=timestamp(0 s since 1904-01-01), "dt"=1.0, "Y"=[]} ("Waveform")
          w468 = "Proc1" ("이름(이름없음)")
          w467 = "Proc0" ("이름(이름없음)")
          w466 = dbl[][] []
          w514 = "SIG0" ("이름(이름없음)")
          w521 = waveform(dbl) {"t0"=timestamp(0 s since 1904-01-01), "dt"=1.0, "Y"=[]} ("Waveform")
          w505 = "SIG1" ("이름(이름없음)")
          w537 = 10123 items=["유한 샘플"=10178, "연속 샘플"=10123, "하드웨어 타이밍에 의한 단일 포인트"=12522] ("sample mode")
          w541 = 10178 items=["유한 샘플"=10178, "연속 샘플"=10123, "하드웨어 타이밍에 의한 단일 포인트"=12522] ("sample mode")
          # "[Post processing]  1. Queue get : Proc0, Proc1 / 2. Threshold estimation with moving average / 3. Peak and valley detection / 4. Demodulation"
          # "[Rx.time]\nTravel time (1km) : 670ms * 2\nDown-link : 210ms\nUp-link : 1024ms\nTotal : Rx.time > 2574ms"
          # "Local variable"
          # "Queue clear"
          # "[Data Acquistion (ADC)]"
          # "Signal generation (Counter) / delaty time : 200ms"
          # "[Signal processing]\n1. Queue get : SIG0\n2. Data type converting : Waveform (DBL) --> Array (DBL)\n3. DDC (Digital to Digital Convering)\n  - DSB modulation : Multiply carrier signal (30kHz)\n  - Decimate : 192kHz sample rate --> 16kHz sample rate\n4. Cross-correlation with down-chirp (4k ~ 0Hz)\n5. Envelope detection (Hilbert transform) & square\n6. Queue put : Proc1"
          # "[Signal processing]\n1. Queue get : SIG0\n2. Data type converting : Waveform (DBL) --> Array (DBL)\n3. DDC (Digital to Digital Convering)\n  - DSB modulation : Multiply carrier signal (30kHz)\n  - Decimate : 192kHz sample rate --> 16kHz sample rate\n4. Cross-correlation with up-chirp (0 ~ 4kHz)\n5. Envelope detection (Hilbert transform) & square\n6. Queue put : Proc0"
          # "[Data Acquistion (ADC)]\n1. Device reset\n2. Creat channel\n3, Set sample clock\n  - Sampling frequency : 192kHz\n  - Number of sample (Chunk size) : 38400\n4. Start task\n5. Data read\n6. Queue put : SIG0, SIG1\n  - Queue data type : Waveform (DBL)"
          n226 = local read "Number of pulse"() -> (w542:i32)
          n227 = local read "Output terminal"() -> (w545:tag)
          n228 = local read "Sampling freuqncy(Hz)"() -> (w473:dbl)
          n229 = local read "Physical channel"() -> (w539:tag)
          n230 = local read "Frequency(Hz)"() -> (w550:dbl)
          n231 = Build Array(w491, w491, w491, w491, w491, w491, w491, w491) -> (w490:waveform(dbl)[])
          n232 = local read "Cycle share"() -> (w549:dbl)
          n233 = local read "Number of sample"() -> (w472:i32)
          n234 = local read "Counter"() -> (w551:tag)
          n235 = Obtain Queue(name (unnamed)="SIG1" ("이름(이름없음)"), element data type=w490) -> (queue out=w487:refnum<queue>, error out=w486:errorcluster)  [unwired: 3 in, 1 out]
          n236 = Obtain Queue(name (unnamed)="Proc1" ("이름(이름없음)"), element data type=w475) -> (queue out=w479:refnum<queue>, error out=w478:errorcluster)  [unwired: 3 in, 1 out]
          n237 = Obtain Queue(name (unnamed)="SIG0" ("이름(이름없음)"), element data type=w490) -> (queue out=w497:refnum<queue>, error out=w496:errorcluster)  [unwired: 3 in, 1 out]
          n238 = Obtain Queue(name (unnamed)="Proc0" ("이름(이름없음)"), element data type=w475) -> (queue out=w485:refnum<queue>, error out=w484:errorcluster)  [unwired: 3 in, 1 out]
          n239 = call-poly <vilib>:"DAQmx Create Virtual Channel.vi"("frequency"=w550, "duty cycle"=w549, "counter"=w551, "error in"=w548) -> ("task out"=w547:refnum<k21>, "error out"=w546:errorcluster)  [unwired: 10 in]
          n240 = call-poly <vilib>:"DAQmx Create Virtual Channel.vi"("physical channels"=w539) -> ("task out"=w538:refnum<k21>, "error out"=w540:errorcluster)  [unwired: 8 in, 5 out]
          n241 = Flush Queue(queue=w497, error in (no error)=w496) -> (queue out=w495:refnum<queue>, error out=w494:errorcluster)  [unwired: 1 out]
          n242 = Flush Queue(queue=w487, error in (no error)=w486) -> (queue out=w489:refnum<queue>, error out=w488:errorcluster)  [unwired: 1 out]
          n243 = Flush Queue(queue=w485, error in (no error)=w484) -> (queue out=w483:refnum<queue>, error out=w482:errorcluster)  [unwired: 1 out]
          n244 = Flush Queue(queue=w479, error in (no error)=w478) -> (queue out=w481:refnum<queue>, error out=w480:errorcluster)  [unwired: 1 out]
          n245 = property class="DAQmx 채널"(reference=w547, error in=w546, "CO.Pulse.Term"=w545) -> (reference out=w544:refnum<k21>, error out=w543:errorcluster)
          n246 = Release Queue(queue=w495, error in (no error)=w494) -> ()  [unwired: 1 in, 3 out]
          n247 = Release Queue(queue=w489, error in (no error)=w488) -> ()  [unwired: 1 in, 3 out]
          n248 = Release Queue(queue=w483, error in (no error)=w482) -> ()  [unwired: 1 in, 3 out]
          n249 = Release Queue(queue=w481, error in (no error)=w480) -> ()  [unwired: 1 in, 3 out]
          n250 = call-poly <vilib>:"DAQmx Timing.vi"("task/channels in"=w538, "sample mode"=w537, "samples per channel"=w472, "rate"=w473, "error in"=w540) -> ("task out"=w536:refnum<k21>, "error out"=w535:errorcluster)  [unwired: 2 in, 7 out]
          n251 = call-poly <vilib>:"DAQmx Timing.vi"("task/channels in"=w544, "sample mode"=w541, "samples per channel"=w542, "error in"=w543) -> ("task out"=w534:refnum<k21>, "error out"=w533:errorcluster)  [unwired: 10 in]
          n252 = flat-sequence {
            tunnel: w536 -> [w889]
            tunnel: w535 -> [w888]
            tunnel: w534 -> [w887]
            tunnel: w533 -> [w886]
            tunnel: [w887] -> w532
            tunnel: [w886] -> w531
            tunnel: [w885] -> w503
            tunnel: [w884] -> w502
            frame #0 {
              n253 = call <vilib>:"DAQmx Start Task.vi"("task/channels in"=w889, "error in"=w888) -> ("task out"=w885:refnum<k21>, "error out"=w884:errorcluster)  [unwired: 12 in]
            }
          }
          n254 = for {
            N: 2 -> [_]
            tunnel: w532 -> [w882]
            tunnel: [w877] -> w529
            tunnel: w531 -> [w883]
            tunnel: [w876] -> w528
            n255 = call <vilib>:"DAQmx Start Task.vi"("task/channels in"=w882, "error in"=w883) -> ("task out"=w881:refnum<k21>, "error out"=w880:errorcluster)  [unwired: 12 in]
            n256 = call <vilib>:"DAQmx Is Task Done.vi"("task/channels in"=w881, "error in"=w880) -> ("task out"=w879:refnum<k21>, "error out"=w878:errorcluster)  [unwired: 11 in, 1 out]
            n257 = Wait (ms)(milliseconds to wait=u32 200 ("대기 시간 (ms)")) -> ()  [unwired: 1 out]
            n258 = call <vilib>:"DAQmx Stop Task.vi"("task/channels in"=w879, "error in"=w878) -> ("task out"=w877:refnum<k21>, "error out"=w876:errorcluster)  [unwired: 12 in]
          }
          n259 = Multiply(x=3.0, y=w473) -> (x*y=w471:dbl)
          n260 = To Double Precision Float(number=w472) -> (double precision float=w470:dbl)
          n261 = Divide(x=w471, y=w470) -> (x/y=w469:dbl)
          n262 = To Long Integer(number=w469) -> (32bit integer=w457:i32)
          n263 = call <vilib>:"DAQmx Clear Task.vi"("task in"=w529, "error in"=w528) -> ()  [unwired: 13 in, 1 out]
          n264 = Build Array(w521, w521, w521, w521, w521, w521, w521, w521) -> (w504:waveform(dbl)[])
          n265 = Obtain Queue(name (unnamed)=w505, element data type=w504) -> (queue out=w523:refnum<queue>, error out=w522:errorcluster)  [unwired: 3 in, 1 out]
          n266 = Obtain Queue(name (unnamed)=w514, element data type=w504) -> (queue out=w520:refnum<queue>, error out=w519:errorcluster)  [unwired: 3 in, 1 out]
          n267 = for {
            N: w457 -> [_]
            tunnel: w503 -> [w874]
            tunnel: w502 -> [w873]
            tunnel: [w872] -> w526
            tunnel: [w871] -> w527
            tunnel: w472 -> [w870]
            tunnel: w523 -> [w869]
            tunnel: w522 -> [w868]
            tunnel: w520 -> [w867]
            tunnel: w519 -> [w866]
            i -> [w864]
            n268 = call-poly <vilib>:"DAQmx Read.vi"("task/channels in"=w874, "number of samples per channel"=w870, "error in"=w873) -> ("task out"=w872:refnum<k21>, "data"=w865:waveform(dbl)[], "error out"=w871:errorcluster)  [unwired: 10 out]
            n269 = Enqueue Element(queue=w867, element=w865, error in (no error)=w866) -> ()  [unwired: 1 in, 3 out]
            n270 = Enqueue Element(queue=w869, element=w865, error in (no error)=w868) -> ()  [unwired: 1 in, 3 out]
            "숫자형 5" <- w864
          }
          n271 = local read "Decimation rate"() -> (w500:i32)
          n272 = local read "Coefficient_bit0"() -> (w499:dbl[])
          n273 = local read "Coefficient_bit1"() -> (w498:dbl[])
          n274 = local read "MovingAvrParm"() -> (w461:dbl[])
          n275 = local read "ThresholdMargin"() -> (w460:dbl)
          n276 = local read "Deci_Chunk"() -> (w459:i32)
          n277 = local read "Target code"() -> (w458:dbl[])
          n278 = local read "Carrier signal"() -> (w501:dbl[])
          n279 = call <vilib>:"DAQmx Stop Task.vi"("task/channels in"=w526, "error in"=w527) -> ("task out"=w525:refnum<k21>, "error out"=w524:errorcluster)  [unwired: 12 out]
          n280 = call <vilib>:"DAQmx Clear Task.vi"("task in"=w525, "error in"=w524) -> ()  [unwired: 14 out]
          n281 = Obtain Queue(name (unnamed)=w467, element data type=w466) -> (queue out=w518:refnum<queue>, error out=w517:errorcluster)  [unwired: 3 in, 1 out]
          n282 = Obtain Queue(name (unnamed)=w514, element data type=w504) -> (queue out=w516:refnum<queue>, error out=w515:errorcluster)  [unwired: 3 in, 1 out]
          n283 = for {
            N: w457 -> [_]
            tunnel: w516 -> [w863]
            tunnel: w515 -> [w862]
            tunnel: w518 -> [w861]
            tunnel: w517 -> [w860]
            tunnel: [w859] -> w513
            tunnel: [w858] -> w512
            tunnel: w501 -> [w798]
            tunnel: w500 -> [w797]
            tunnel: w499 -> [w796]
            i -> [w794]
            w808 = TRUE ("averaging")
            w857 = TRUE ("init/cont (init:F)")
            n284 = Dequeue Element(queue=w863, error in (no error)=w862) -> (queue out=w859:refnum<queue>, element=w799:waveform(dbl)[], error out=w858:errorcluster)  [unwired: 2 out]
            n285 = Index Array(array=w799) -> (element #1=w856:waveform(dbl), element #2=w855:waveform(dbl), element #3=w854:waveform(dbl), element #4=w853:waveform(dbl), element #5=w852:waveform(dbl), element #6=w851:waveform(dbl), element #7=w850:waveform(dbl), element #8=w849:waveform(dbl))  [unwired: 8 in]
            n286 = Unbundle By Name(w856) -> ("Y"=w848:dbl[])
            n287 = Unbundle By Name(w855) -> ("Y"=w847:dbl[])
            n288 = Unbundle By Name(w854) -> ("Y"=w846:dbl[])
            n289 = Unbundle By Name(w853) -> ("Y"=w845:dbl[])
            n290 = Unbundle By Name(w852) -> ("Y"=w844:dbl[])
            n291 = Unbundle By Name(w851) -> ("Y"=w843:dbl[])
            n292 = Unbundle By Name(w850) -> ("Y"=w842:dbl[])
            n293 = Unbundle By Name(w849) -> ("Y"=w841:dbl[])
            n294 = Multiply(x=w848, y=w798) -> (x*y=w823:dbl[])
            n295 = Multiply(x=w847, y=w798) -> (x*y=w822:dbl[])
            n296 = Multiply(x=w846, y=w798) -> (x*y=w821:dbl[])
            n297 = Multiply(x=w845, y=w798) -> (x*y=w820:dbl[])
            n298 = Multiply(x=w844, y=w798) -> (x*y=w819:dbl[])
            n299 = Multiply(x=w843, y=w798) -> (x*y=w818:dbl[])
            n300 = Multiply(x=w842, y=w798) -> (x*y=w817:dbl[])
            n301 = Multiply(x=w841, y=w798) -> (x*y=w816:dbl[])
            n302 = call-poly <vilib>:"Decimate (single shot).vi"("averaging"=w808, "decimating factor"=w797, "X"=w818) -> ("Decimated Array"=w811:dbl[])  [unwired: 7 in, 1 out]
            n303 = call-poly <vilib>:"Decimate (single shot).vi"("averaging"=w808, "decimating factor"=w797, "X"=w816) -> ("Decimated Array"=w809:dbl[])  [unwired: 7 in, 1 out]
            n304 = call-poly <vilib>:"Decimate (single shot).vi"("averaging"=w808, "decimating factor"=w797, "X"=w822) -> ("Decimated Array"=w815:dbl[])  [unwired: 7 in, 1 out]
            n305 = call-poly <vilib>:"Decimate (single shot).vi"("averaging"=w808, "decimating factor"=w797, "X"=w820) -> ("Decimated Array"=w813:dbl[])  [unwired: 7 in, 1 out]
            n306 = call-poly <vilib>:"Decimate (single shot).vi"("averaging"=w808, "decimating factor"=w797, "X"=w819) -> ("Decimated Array"=w812:dbl[])  [unwired: 7 in, 1 out]
            n307 = call-poly <vilib>:"Decimate (single shot).vi"("averaging"=w808, "decimating factor"=w797, "X"=w817) -> ("Decimated Array"=w810:dbl[])  [unwired: 7 in, 1 out]
            n308 = call-poly <vilib>:"Decimate (single shot).vi"("averaging"=w808, "decimating factor"=w797, "X"=w823) -> ("Decimated Array"=w824:dbl[])  [unwired: 7 in, 1 out]
            n309 = call-poly <vilib>:"Decimate (single shot).vi"("averaging"=w808, "decimating factor"=w797, "X"=w821) -> ("Decimated Array"=w814:dbl[])  [unwired: 7 in, 1 out]
            n310 = call-poly <vilib>:"FIR Filter.vi"("init/cont (init:F)"=w857, "FIR Coefficients"=w796, "X"=w824) -> ("Filtered X"=w840:dbl[])  [unwired: 1 in, 1 out]
            n311 = call-poly <vilib>:"FIR Filter.vi"("init/cont (init:F)"=w857, "FIR Coefficients"=w796, "X"=w815) -> ("Filtered X"=w839:dbl[])  [unwired: 1 in, 1 out]
            n312 = call-poly <vilib>:"FIR Filter.vi"("init/cont (init:F)"=w857, "FIR Coefficients"=w796, "X"=w814) -> ("Filtered X"=w838:dbl[])  [unwired: 1 in, 1 out]
            n313 = call-poly <vilib>:"FIR Filter.vi"("init/cont (init:F)"=w857, "FIR Coefficients"=w796, "X"=w813) -> ("Filtered X"=w837:dbl[])  [unwired: 1 in, 1 out]
            n314 = call-poly <vilib>:"FIR Filter.vi"("init/cont (init:F)"=w857, "FIR Coefficients"=w796, "X"=w812) -> ("Filtered X"=w836:dbl[])  [unwired: 1 in, 1 out]
            n315 = call-poly <vilib>:"FIR Filter.vi"("init/cont (init:F)"=w857, "FIR Coefficients"=w796, "X"=w811) -> ("Filtered X"=w835:dbl[])  [unwired: 1 in, 1 out]
            n316 = call-poly <vilib>:"FIR Filter.vi"("init/cont (init:F)"=w857, "FIR Coefficients"=w796, "X"=w810) -> ("Filtered X"=w834:dbl[])  [unwired: 1 in, 1 out]
            n317 = call-poly <vilib>:"FIR Filter.vi"("init/cont (init:F)"=w857, "FIR Coefficients"=w796, "X"=w809) -> ("Filtered X"=w833:dbl[])  [unwired: 1 in, 1 out]
            n318 = call "Envelope(SubVI).vi"("x"=w840) -> ("Y"=w832:dbl[])
            n319 = call "Envelope(SubVI).vi"("x"=w839) -> ("Y"=w831:dbl[])
            n320 = call "Envelope(SubVI).vi"("x"=w838) -> ("Y"=w830:dbl[])
            n321 = call "Envelope(SubVI).vi"("x"=w837) -> ("Y"=w829:dbl[])
            n322 = call "Envelope(SubVI).vi"("x"=w836) -> ("Y"=w828:dbl[])
            n323 = call "Envelope(SubVI).vi"("x"=w835) -> ("Y"=w827:dbl[])
            n324 = call "Envelope(SubVI).vi"("x"=w834) -> ("Y"=w826:dbl[])
            n325 = call "Envelope(SubVI).vi"("x"=w833) -> ("Y"=w825:dbl[])
            n326 = Square(x=w832) -> (x^2=w807:dbl[])
            n327 = Square(x=w831) -> (x^2=w806:dbl[])
            n328 = Square(x=w830) -> (x^2=w805:dbl[])
            n329 = Square(x=w829) -> (x^2=w804:dbl[])
            n330 = Square(x=w828) -> (x^2=w803:dbl[])
            n331 = Square(x=w827) -> (x^2=w802:dbl[])
            n332 = Square(x=w826) -> (x^2=w801:dbl[])
            n333 = Square(x=w825) -> (x^2=w800:dbl[])
            n334 = Build Array(w807, w806, w805, w804, w803, w802, w801, w800) -> (w795:dbl[][])
            n335 = Enqueue Element(queue=w861, element=w795, error in (no error)=w860) -> ()  [unwired: 1 in, 3 out]
            "숫자형 6" <- w794
          }
          n336 = Release Queue(queue=w513, error in (no error)=w512) -> ()  [unwired: 1 in, 3 out]
          n337 = Obtain Queue(name (unnamed)=w468, element data type=w466) -> (queue out=w511:refnum<queue>, error out=w510:errorcluster)  [unwired: 3 in, 1 out]
          n338 = Obtain Queue(name (unnamed)=w505, element data type=w504) -> (queue out=w509:refnum<queue>, error out=w508:errorcluster)  [unwired: 3 in, 1 out]
          n339 = for {
            N: w457 -> [_]
            tunnel: w509 -> [w793]
            tunnel: w508 -> [w792]
            tunnel: w511 -> [w791]
            tunnel: w510 -> [w790]
            tunnel: [w789] -> w507
            tunnel: [w788] -> w506
            tunnel: w501 -> [w728]
            tunnel: w500 -> [w727]
            tunnel: w498 -> [w726]
            i -> [w724]
            w738 = TRUE ("averaging")
            w787 = TRUE ("init/cont (init:F)")
            n340 = Dequeue Element(queue=w793, error in (no error)=w792) -> (queue out=w789:refnum<queue>, element=w729:waveform(dbl)[], error out=w788:errorcluster)  [unwired: 2 out]
            n341 = Index Array(array=w729) -> (element #1=w786:waveform(dbl), element #2=w785:waveform(dbl), element #3=w784:waveform(dbl), element #4=w783:waveform(dbl), element #5=w782:waveform(dbl), element #6=w781:waveform(dbl), element #7=w780:waveform(dbl), element #8=w779:waveform(dbl))  [unwired: 8 in]
            n342 = Unbundle By Name(w786) -> ("Y"=w778:dbl[])
            n343 = Unbundle By Name(w785) -> ("Y"=w777:dbl[])
            n344 = Unbundle By Name(w784) -> ("Y"=w776:dbl[])
            n345 = Unbundle By Name(w783) -> ("Y"=w775:dbl[])
            n346 = Unbundle By Name(w782) -> ("Y"=w774:dbl[])
            n347 = Unbundle By Name(w781) -> ("Y"=w773:dbl[])
            n348 = Unbundle By Name(w780) -> ("Y"=w772:dbl[])
            n349 = Unbundle By Name(w779) -> ("Y"=w771:dbl[])
            n350 = Multiply(x=w778, y=w728) -> (x*y=w753:dbl[])
            n351 = Multiply(x=w777, y=w728) -> (x*y=w752:dbl[])
            n352 = Multiply(x=w776, y=w728) -> (x*y=w751:dbl[])
            n353 = Multiply(x=w775, y=w728) -> (x*y=w750:dbl[])
            n354 = Multiply(x=w774, y=w728) -> (x*y=w749:dbl[])
            n355 = Multiply(x=w773, y=w728) -> (x*y=w748:dbl[])
            n356 = Multiply(x=w772, y=w728) -> (x*y=w747:dbl[])
            n357 = Multiply(x=w771, y=w728) -> (x*y=w746:dbl[])
            n358 = call-poly <vilib>:"Decimate (single shot).vi"("averaging"=w738, "decimating factor"=w727, "X"=w748) -> ("Decimated Array"=w741:dbl[])  [unwired: 7 in, 1 out]
            n359 = call-poly <vilib>:"Decimate (single shot).vi"("averaging"=w738, "decimating factor"=w727, "X"=w746) -> ("Decimated Array"=w739:dbl[])  [unwired: 7 in, 1 out]
            n360 = call-poly <vilib>:"Decimate (single shot).vi"("averaging"=w738, "decimating factor"=w727, "X"=w752) -> ("Decimated Array"=w745:dbl[])  [unwired: 7 in, 1 out]
            n361 = call-poly <vilib>:"Decimate (single shot).vi"("averaging"=w738, "decimating factor"=w727, "X"=w750) -> ("Decimated Array"=w743:dbl[])  [unwired: 7 in, 1 out]
            n362 = call-poly <vilib>:"Decimate (single shot).vi"("averaging"=w738, "decimating factor"=w727, "X"=w749) -> ("Decimated Array"=w742:dbl[])  [unwired: 7 in, 1 out]
            n363 = call-poly <vilib>:"Decimate (single shot).vi"("averaging"=w738, "decimating factor"=w727, "X"=w747) -> ("Decimated Array"=w740:dbl[])  [unwired: 7 in, 1 out]
            n364 = call-poly <vilib>:"Decimate (single shot).vi"("averaging"=w738, "decimating factor"=w727, "X"=w753) -> ("Decimated Array"=w754:dbl[])  [unwired: 7 in, 1 out]
            n365 = call-poly <vilib>:"Decimate (single shot).vi"("averaging"=w738, "decimating factor"=w727, "X"=w751) -> ("Decimated Array"=w744:dbl[])  [unwired: 7 in, 1 out]
            n366 = call-poly <vilib>:"FIR Filter.vi"("init/cont (init:F)"=w787, "FIR Coefficients"=w726, "X"=w754) -> ("Filtered X"=w770:dbl[])  [unwired: 1 in, 1 out]
            n367 = call-poly <vilib>:"FIR Filter.vi"("init/cont (init:F)"=w787, "FIR Coefficients"=w726, "X"=w745) -> ("Filtered X"=w769:dbl[])  [unwired: 1 in, 1 out]
            n368 = call-poly <vilib>:"FIR Filter.vi"("init/cont (init:F)"=w787, "FIR Coefficients"=w726, "X"=w744) -> ("Filtered X"=w768:dbl[])  [unwired: 1 in, 1 out]
            n369 = call-poly <vilib>:"FIR Filter.vi"("init/cont (init:F)"=w787, "FIR Coefficients"=w726, "X"=w743) -> ("Filtered X"=w767:dbl[])  [unwired: 1 in, 1 out]
            n370 = call-poly <vilib>:"FIR Filter.vi"("init/cont (init:F)"=w787, "FIR Coefficients"=w726, "X"=w742) -> ("Filtered X"=w766:dbl[])  [unwired: 1 in, 1 out]
            n371 = call-poly <vilib>:"FIR Filter.vi"("init/cont (init:F)"=w787, "FIR Coefficients"=w726, "X"=w741) -> ("Filtered X"=w765:dbl[])  [unwired: 1 in, 1 out]
            n372 = call-poly <vilib>:"FIR Filter.vi"("init/cont (init:F)"=w787, "FIR Coefficients"=w726, "X"=w740) -> ("Filtered X"=w764:dbl[])  [unwired: 1 in, 1 out]
            n373 = call-poly <vilib>:"FIR Filter.vi"("init/cont (init:F)"=w787, "FIR Coefficients"=w726, "X"=w739) -> ("Filtered X"=w763:dbl[])  [unwired: 1 in, 1 out]
            n374 = call "Envelope(SubVI).vi"("x"=w770) -> ("Y"=w762:dbl[])
            n375 = call "Envelope(SubVI).vi"("x"=w769) -> ("Y"=w761:dbl[])
            n376 = call "Envelope(SubVI).vi"("x"=w768) -> ("Y"=w760:dbl[])
            n377 = call "Envelope(SubVI).vi"("x"=w767) -> ("Y"=w759:dbl[])
            n378 = call "Envelope(SubVI).vi"("x"=w766) -> ("Y"=w758:dbl[])
            n379 = call "Envelope(SubVI).vi"("x"=w765) -> ("Y"=w757:dbl[])
            n380 = call "Envelope(SubVI).vi"("x"=w764) -> ("Y"=w756:dbl[])
            n381 = call "Envelope(SubVI).vi"("x"=w763) -> ("Y"=w755:dbl[])
            n382 = Square(x=w762) -> (x^2=w737:dbl[])
            n383 = Square(x=w761) -> (x^2=w736:dbl[])
            n384 = Square(x=w760) -> (x^2=w735:dbl[])
            n385 = Square(x=w759) -> (x^2=w734:dbl[])
            n386 = Square(x=w758) -> (x^2=w733:dbl[])
            n387 = Square(x=w757) -> (x^2=w732:dbl[])
            n388 = Square(x=w756) -> (x^2=w731:dbl[])
            n389 = Square(x=w755) -> (x^2=w730:dbl[])
            n390 = Build Array(w737, w736, w735, w734, w733, w732, w731, w730) -> (w725:dbl[][])
            n391 = Enqueue Element(queue=w791, element=w725, error in (no error)=w790) -> ()  [unwired: 1 in, 3 out]
            "숫자형 7" <- w724
          }
          n392 = Release Queue(queue=w507, error in (no error)=w506) -> ()  [unwired: 1 in, 3 out]
          n393 = Obtain Queue(name (unnamed)=w467, element data type=w466) -> (queue out=w465:refnum<queue>, error out=w464:errorcluster)  [unwired: 3 in, 1 out]
          n394 = Obtain Queue(name (unnamed)=w468, element data type=w466) -> (queue out=w463:refnum<queue>, error out=w462:errorcluster)  [unwired: 3 in, 1 out]
          n395 = for {
            N: w457 -> [_]
            tunnel: w465 -> [w723]
            tunnel: w464 -> [w722]
            tunnel: w463 -> [w721]
            tunnel: w462 -> [w720]
            tunnel: w461 -> [w718]
            tunnel: w460 -> [w682]
            tunnel: [w662] -> _
            tunnel: [w661] -> _
            tunnel: [w660] -> _
            tunnel: [w659] -> _
            tunnel: w458 -> [w658]
            shift-right: [w584] -> _
            shift-left: w456 -> [w607]
            shift-right: [w585] -> _
            shift-left: w456 -> [w606]
            shift-right: [w586] -> _
            shift-left: w456 -> [w605]
            shift-right: [w587] -> _
            shift-left: w456 -> [w604]
            shift-right: [w588] -> _
            shift-left: w456 -> [w603]
            shift-right: [w589] -> _
            shift-left: w456 -> [w602]
            shift-right: [w590] -> _
            shift-left: w456 -> [w601]
            shift-right: [w591] -> _
            shift-left: w456 -> [w600]
            tunnel: w459 -> [w625]
            shift-right: [w559] -> w455
            shift-left: w447 -> [w567]
            shift-right: [w552] -> w454
            shift-left: w447 -> [w566]
            shift-right: [w553] -> w453
            shift-left: w447 -> [w565]
            shift-right: [w554] -> w452
            shift-left: w447 -> [w564]
            shift-right: [w555] -> w451
            shift-left: w447 -> [w563]
            shift-right: [w556] -> w450
            shift-left: w447 -> [w562]
            shift-right: [w557] -> w449
            shift-left: w447 -> [w561]
            shift-right: [w558] -> w448
            shift-left: w447 -> [w560]
            i -> [w624]
            w707 = enum32{"Peaks", "Valleys"}."Valleys" ("peaks/valleys")
            w708 = enum32{"Peaks", "Valleys"}."Peaks" ("peaks/valleys")
            w706 = 5 ("width")
            w717 = TRUE ("init/cont (init:F)")
            n396 = Dequeue Element(queue=w723, error in (no error)=w722) -> (queue out=w662:refnum<queue>, element=w664:dbl[][], error out=w661:errorcluster)  [unwired: 2 out]
            n397 = Dequeue Element(queue=w721, error in (no error)=w720) -> (queue out=w660:refnum<queue>, element=w663:dbl[][], error out=w659:errorcluster)  [unwired: 2 out]
            n398 = Subtract(x=w664, y=w663) -> (x-y=w719:dbl[][])
            n399 = Index Array(array=w719) -> (element #1=w705:dbl[], element #2=w704:dbl[], element #3=w703:dbl[], element #4=w702:dbl[], element #5=w701:dbl[], element #6=w700:dbl[], element #7=w699:dbl[], element #8=w667:dbl[])  [unwired: 16 in]
            n400 = call-poly <vilib>:"FIR Filter.vi"("init/cont (init:F)"=w717, "FIR Coefficients"=w718, "X"=w705) -> ("Filtered X"=w716:dbl[])  [unwired: 1 in, 1 out]
            n401 = call-poly <vilib>:"FIR Filter.vi"("init/cont (init:F)"=w717, "FIR Coefficients"=w718, "X"=w704) -> ("Filtered X"=w715:dbl[])  [unwired: 1 in, 1 out]
            n402 = call-poly <vilib>:"FIR Filter.vi"("init/cont (init:F)"=w717, "FIR Coefficients"=w718, "X"=w703) -> ("Filtered X"=w714:dbl[])  [unwired: 1 in, 1 out]
            n403 = call-poly <vilib>:"FIR Filter.vi"("init/cont (init:F)"=w717, "FIR Coefficients"=w718, "X"=w702) -> ("Filtered X"=w713:dbl[])  [unwired: 1 in, 1 out]
            n404 = call-poly <vilib>:"FIR Filter.vi"("init/cont (init:F)"=w717, "FIR Coefficients"=w718, "X"=w701) -> ("Filtered X"=w712:dbl[])  [unwired: 1 in, 1 out]
            n405 = call-poly <vilib>:"FIR Filter.vi"("init/cont (init:F)"=w717, "FIR Coefficients"=w718, "X"=w700) -> ("Filtered X"=w711:dbl[])  [unwired: 1 in, 1 out]
            n406 = call-poly <vilib>:"FIR Filter.vi"("init/cont (init:F)"=w717, "FIR Coefficients"=w718, "X"=w699) -> ("Filtered X"=w710:dbl[])  [unwired: 1 in, 1 out]
            n407 = call-poly <vilib>:"FIR Filter.vi"("init/cont (init:F)"=w717, "FIR Coefficients"=w718, "X"=w667) -> ("Filtered X"=w709:dbl[])  [unwired: 1 in, 1 out]
            n408 = Array Max & Min(array=w716) -> (max value=w698:dbl, min value=w697:dbl)  [unwired: 2 out]
            n409 = Array Max & Min(array=w715) -> (max value=w696:dbl, min value=w695:dbl)  [unwired: 2 out]
            n410 = Array Max & Min(array=w714) -> (max value=w694:dbl, min value=w693:dbl)  [unwired: 2 out]
            n411 = Array Max & Min(array=w713) -> (max value=w692:dbl, min value=w691:dbl)  [unwired: 2 out]
            n412 = Array Max & Min(array=w712) -> (max value=w690:dbl, min value=w689:dbl)  [unwired: 2 out]
            n413 = Array Max & Min(array=w711) -> (max value=w688:dbl, min value=w687:dbl)  [unwired: 2 out]
            n414 = Array Max & Min(array=w710) -> (max value=w686:dbl, min value=w685:dbl)  [unwired: 2 out]
            n415 = Array Max & Min(array=w709) -> (max value=w684:dbl, min value=w683:dbl)  [unwired: 2 out]
            n416 = call "ThresholdEstimation(SubVI).vi"("Margin"=w682, "최소값"=w695, "최대값"=w696) -> ("N.Th"=w669:dbl, "P.Th"=w680:dbl)
            n417 = call "ThresholdEstimation(SubVI).vi"("Margin"=w682, "최소값"=w693, "최대값"=w694) -> ("N.Th"=w670:dbl, "P.Th"=w679:dbl)
            n418 = call "ThresholdEstimation(SubVI).vi"("Margin"=w682, "최소값"=w691, "최대값"=w692) -> ("N.Th"=w671:dbl, "P.Th"=w678:dbl)
            n419 = call "ThresholdEstimation(SubVI).vi"("Margin"=w682, "최소값"=w689, "최대값"=w690) -> ("N.Th"=w672:dbl, "P.Th"=w677:dbl)
            n420 = call "ThresholdEstimation(SubVI).vi"("Margin"=w682, "최소값"=w697, "최대값"=w698) -> ("N.Th"=w668:dbl, "P.Th"=w681:dbl)
            n421 = call "ThresholdEstimation(SubVI).vi"("Margin"=w682, "최소값"=w687, "최대값"=w688) -> ("N.Th"=w673:dbl, "P.Th"=w676:dbl)
            n422 = call "ThresholdEstimation(SubVI).vi"("Margin"=w682, "최소값"=w685, "최대값"=w686) -> ("N.Th"=w674:dbl, "P.Th"=w675:dbl)
            n423 = call "ThresholdEstimation(SubVI).vi"("Margin"=w682, "최소값"=w683, "최대값"=w684) -> ("N.Th"=w666:dbl, "P.Th"=w665:dbl)
            n424 = call <vilib>:"Peak Detector.vi"("peaks/valleys"=w708, "width"=w706, "threshold"=w681, "X"=w705) -> ("Locations"=w655:dbl[], "# found"=w657:i32)  [unwired: 3 in, 3 out]
            n425 = call <vilib>:"Peak Detector.vi"("peaks/valleys"=w708, "width"=w706, "threshold"=w680, "X"=w704) -> ("Locations"=w651:dbl[], "# found"=w653:i32)  [unwired: 3 in, 3 out]
            n426 = call <vilib>:"Peak Detector.vi"("peaks/valleys"=w708, "width"=w706, "threshold"=w679, "X"=w703) -> ("Locations"=w647:dbl[], "# found"=w649:i32)  [unwired: 3 in, 3 out]
            n427 = call <vilib>:"Peak Detector.vi"("peaks/valleys"=w708, "width"=w706, "threshold"=w678, "X"=w702) -> ("Locations"=w643:dbl[], "# found"=w645:i32)  [unwired: 3 in, 3 out]
            n428 = call <vilib>:"Peak Detector.vi"("peaks/valleys"=w708, "width"=w706, "threshold"=w677, "X"=w701) -> ("Locations"=w639:dbl[], "# found"=w641:i32)  [unwired: 3 in, 3 out]
            n429 = call <vilib>:"Peak Detector.vi"("peaks/valleys"=w708, "width"=w706, "threshold"=w676, "X"=w700) -> ("Locations"=w635:dbl[], "# found"=w637:i32)  [unwired: 3 in, 3 out]
            n430 = call <vilib>:"Peak Detector.vi"("peaks/valleys"=w708, "width"=w706, "threshold"=w675, "X"=w699) -> ("Locations"=w631:dbl[], "# found"=w633:i32)  [unwired: 3 in, 3 out]
            n431 = call <vilib>:"Peak Detector.vi"("peaks/valleys"=w708, "width"=w706, "threshold"=w665, "X"=w667) -> ("Locations"=w627:dbl[], "# found"=w629:i32)  [unwired: 3 in, 3 out]
            n432 = call <vilib>:"Peak Detector.vi"("peaks/valleys"=w707, "width"=w706, "threshold"=w668, "X"=w705) -> ("Locations"=w654:dbl[], "# found"=w656:i32)  [unwired: 3 in, 3 out]
            n433 = call <vilib>:"Peak Detector.vi"("peaks/valleys"=w707, "width"=w706, "threshold"=w669, "X"=w704) -> ("Locations"=w650:dbl[], "# found"=w652:i32)  [unwired: 3 in, 3 out]
            n434 = call <vilib>:"Peak Detector.vi"("peaks/valleys"=w707, "width"=w706, "threshold"=w670, "X"=w703) -> ("Locations"=w646:dbl[], "# found"=w648:i32)  [unwired: 3 in, 3 out]
            n435 = call <vilib>:"Peak Detector.vi"("peaks/valleys"=w707, "width"=w706, "threshold"=w671, "X"=w702) -> ("Locations"=w642:dbl[], "# found"=w644:i32)  [unwired: 3 in, 3 out]
            n436 = call <vilib>:"Peak Detector.vi"("peaks/valleys"=w707, "width"=w706, "threshold"=w672, "X"=w701) -> ("Locations"=w638:dbl[], "# found"=w640:i32)  [unwired: 3 in, 3 out]
            n437 = call <vilib>:"Peak Detector.vi"("peaks/valleys"=w707, "width"=w706, "threshold"=w673, "X"=w700) -> ("Locations"=w634:dbl[], "# found"=w636:i32)  [unwired: 3 in, 3 out]
            n438 = call <vilib>:"Peak Detector.vi"("peaks/valleys"=w707, "width"=w706, "threshold"=w674, "X"=w699) -> ("Locations"=w630:dbl[], "# found"=w632:i32)  [unwired: 3 in, 3 out]
            n439 = call <vilib>:"Peak Detector.vi"("peaks/valleys"=w707, "width"=w706, "threshold"=w666, "X"=w667) -> ("Locations"=w626:dbl[], "# found"=w628:i32)  [unwired: 3 in, 3 out]
            n440 = call "Decision2(SubVI).vi"("L_ind0"=w657, "number of sample"=w625, "L_ind1"=w656, "Peak_ind0"=w655, "index"=w624, "Peak_ind1"=w654) -> ("L_sum"=w592:i32, "Bits"=w623:dbl[], "Position"=w622:dbl[])
            n441 = call "Decision2(SubVI).vi"("L_ind0"=w653, "number of sample"=w625, "L_ind1"=w652, "Peak_ind0"=w651, "index"=w624, "Peak_ind1"=w650) -> ("L_sum"=w593:i32, "Bits"=w621:dbl[], "Position"=w620:dbl[])
            n442 = call "Decision2(SubVI).vi"("L_ind0"=w649, "number of sample"=w625, "L_ind1"=w648, "Peak_ind0"=w647, "index"=w624, "Peak_ind1"=w646) -> ("L_sum"=w594:i32, "Bits"=w619:dbl[], "Position"=w618:dbl[])
            n443 = call "Decision2(SubVI).vi"("L_ind0"=w645, "number of sample"=w625, "L_ind1"=w644, "Peak_ind0"=w643, "index"=w624, "Peak_ind1"=w642) -> ("L_sum"=w595:i32, "Bits"=w617:dbl[], "Position"=w616:dbl[])
            n444 = call "Decision2(SubVI).vi"("L_ind0"=w641, "number of sample"=w625, "L_ind1"=w640, "Peak_ind0"=w639, "index"=w624, "Peak_ind1"=w638) -> ("L_sum"=w596:i32, "Bits"=w615:dbl[], "Position"=w614:dbl[])
            n445 = call "Decision2(SubVI).vi"("L_ind0"=w637, "number of sample"=w625, "L_ind1"=w636, "Peak_ind0"=w635, "index"=w624, "Peak_ind1"=w634) -> ("L_sum"=w597:i32, "Bits"=w613:dbl[], "Position"=w612:dbl[])
            n446 = call "Decision2(SubVI).vi"("L_ind0"=w633, "number of sample"=w625, "L_ind1"=w632, "Peak_ind0"=w631, "index"=w624, "Peak_ind1"=w630) -> ("L_sum"=w598:i32, "Bits"=w611:dbl[], "Position"=w610:dbl[])
            n447 = call "Decision2(SubVI).vi"("L_ind0"=w629, "number of sample"=w625, "L_ind1"=w628, "Peak_ind0"=w627, "index"=w624, "Peak_ind1"=w626) -> ("L_sum"=w599:i32, "Bits"=w609:dbl[], "Position"=w608:dbl[])
            n448 = call "TImeThresholdLogic(SubVI).vi"("Position"=w622, "Bits"=w623, "Buffer"=w607) -> ("Data"=w584:dbl[][])  [unwired: 1 in]
            n449 = call "TImeThresholdLogic(SubVI).vi"("Position"=w620, "Bits"=w621, "Buffer"=w606) -> ("Data"=w585:dbl[][])  [unwired: 1 in]
            n450 = call "TImeThresholdLogic(SubVI).vi"("Position"=w618, "Bits"=w619, "Buffer"=w605) -> ("Data"=w586:dbl[][])  [unwired: 1 in]
            n451 = call "TImeThresholdLogic(SubVI).vi"("Position"=w616, "Bits"=w617, "Buffer"=w604) -> ("Data"=w587:dbl[][])  [unwired: 1 in]
            n452 = call "TImeThresholdLogic(SubVI).vi"("Position"=w614, "Bits"=w615, "Buffer"=w603) -> ("Data"=w588:dbl[][])  [unwired: 1 in]
            n453 = call "TImeThresholdLogic(SubVI).vi"("Position"=w612, "Bits"=w613, "Buffer"=w602) -> ("Data"=w589:dbl[][])  [unwired: 1 in]
            n454 = call "TImeThresholdLogic(SubVI).vi"("Position"=w610, "Bits"=w611, "Buffer"=w601) -> ("Data"=w590:dbl[][])  [unwired: 1 in]
            n455 = call "TImeThresholdLogic(SubVI).vi"("Position"=w608, "Bits"=w609, "Buffer"=w600) -> ("Data"=w591:dbl[][])  [unwired: 1 in]
            n456 = call "CodeDetection(SubVI).vi"("Code"=w658, "Buff"=w584, "L_sum"=w592) -> ("detect"=w582:bool, "Position"=w583:dbl[])
            n457 = call "CodeDetection(SubVI).vi"("Code"=w658, "Buff"=w585, "L_sum"=w593) -> ("detect"=w580:bool, "Position"=w581:dbl[])
            n458 = call "CodeDetection(SubVI).vi"("Code"=w658, "Buff"=w586, "L_sum"=w594) -> ("detect"=w578:bool, "Position"=w579:dbl[])
            n459 = call "CodeDetection(SubVI).vi"("Code"=w658, "Buff"=w587, "L_sum"=w595) -> ("detect"=w576:bool, "Position"=w577:dbl[])
            n460 = call "CodeDetection(SubVI).vi"("Code"=w658, "Buff"=w588, "L_sum"=w596) -> ("detect"=w574:bool, "Position"=w575:dbl[])
            n461 = call "CodeDetection(SubVI).vi"("Code"=w658, "Buff"=w589, "L_sum"=w597) -> ("detect"=w572:bool, "Position"=w573:dbl[])
            n462 = call "CodeDetection(SubVI).vi"("Code"=w658, "Buff"=w590, "L_sum"=w598) -> ("detect"=w570:bool, "Position"=w571:dbl[])
            n463 = call "CodeDetection(SubVI).vi"("Code"=w658, "Buff"=w591, "L_sum"=w599) -> ("detect"=w568:bool, "Position"=w569:dbl[])
            n464 = call "ValidPosition(SubVI).vi"("detection"=w582, "BUff"=w567, "Postion"=w583) -> ("Valid Position"=w559:dbl[])
            n465 = call "ValidPosition(SubVI).vi"("detection"=w580, "BUff"=w566, "Postion"=w581) -> ("Valid Position"=w552:dbl[])
            n466 = call "ValidPosition(SubVI).vi"("detection"=w578, "BUff"=w565, "Postion"=w579) -> ("Valid Position"=w553:dbl[])
            n467 = call "ValidPosition(SubVI).vi"("detection"=w576, "BUff"=w564, "Postion"=w577) -> ("Valid Position"=w554:dbl[])
            n468 = call "ValidPosition(SubVI).vi"("detection"=w574, "BUff"=w563, "Postion"=w575) -> ("Valid Position"=w555:dbl[])
            n469 = call "ValidPosition(SubVI).vi"("detection"=w572, "BUff"=w562, "Postion"=w573) -> ("Valid Position"=w556:dbl[])
            n470 = call "ValidPosition(SubVI).vi"("detection"=w570, "BUff"=w561, "Postion"=w571) -> ("Valid Position"=w557:dbl[])
            n471 = call "ValidPosition(SubVI).vi"("detection"=w568, "BUff"=w560, "Postion"=w569) -> ("Valid Position"=w558:dbl[])
          }
          "Position 0" <- w455
          "Position 1" <- w454
          "Position 2" <- w453
          "Position 3" <- w452
          "Position 4" <- w451
          "Position 5" <- w450
          "Position 6" <- w449
          "Position 7" <- w448
        }
      }
    }
  }
